vi "Host.vi"() -> ()   [LabVIEW 2018]
uses:
  <vilib>/userdefined/High Color/nirio_resource_hc.ctl
  <instrlib>/niDCPower/nidcpower.llb/niDCPower Measurement Type.ctl
  <vilib>/FPGAPlugInAG/PXI-7953R/niLvFpga_Open_PXI-7953R.vi
  <vilib>/rvi/interface/common/dynamic/niFpgaDynamicAddResources.vi
  <vilib>/FPGAPlugInAG/Dynamic/niLvFpga_Reset_Dynamic.vi
  <vilib>/FPGAPlugInAG/Dynamic/niLvFpga_Run_Dynamic.vi
  <vilib>/Utility/error.llb/Error Cluster From Error Code.vi
  <vilib>/rvi/errors/niLvFpgaAdjustHostInterfaceError.vi
  <vilib>/FPGAPlugInAG/Dynamic/niLvFpga_Abort_Dynamic.vi
  <vilib>/rvi/interface/nirviOpenFPGA/nirviOpenFPGA.xnode
  FPGA Bitfiles/EV76C661_FPGATarget_Target_LxE3WAGXilk.lvbitx
  <vilib>/rvi/interface/nirviMethod/nirviMethod.xnode
  <vilib>/rvi/interface/nirviReadWriteControl/nirviReadWriteControl.xnode
  NiFpgaLv.dll
  <vilib>/rvi/interface/Simulation/niFpgaSimulationCallBeginRW.vi
  <vilib>/FPGAPlugInAG/Dynamic/niLvFpga_ReadFifo_Dynamic.vi
  <vilib>/rvi/errors/niLvFpgaMergeErrorWithErrorCode.vi
panel:
  out "Image":T1(plugin-control)
  in  "Содержание всех регистров":u32[](array[numeric])=[1, 0, 0, 0, 32880, 0, 53338, 2561, 56217, 24976, 512, 260, 0, 0, 512, 0, 0, 0, 6, 1024, 6, 1280, 0, 0, 0, 0, 0, 512, 0, 0, 0, 6, 1024, 6, 1280, 0, 512, 0, 0, 0, 6, 1024, 6, 1280, 0, 512, 0, 0, 0, 6, 1024, 6, 1280, 0, 32896, 32896, 0, 14464, 32960, 0, 0, 0, 0, 0, 0, 0, 0, 0, 8192, 0, 0, 0, 0, 31601, 0, 0, 0, 0, 0, 0, 0, 0, 0, 0, 0, 0, 0, 0, 0, 0, 0, 0, 0, 0, 0, 0, 0, 0, 0, 0, 0, 0, 0, 0, 0, 0, 0, 0, 0, 0, 0, 0, 0, 0, 0, 0, 0, 0, 0, 0, 0, 0, 0, 0, 0, 0, 0, 2048]
  in  "Запись 6 регистров":u32[](array[numeric])=[2561, 56217, 24976, 512, 260, 512]
  in  "SPI_прошить":bool
  out "ST":bool
  in  "RESET":bool
  in  "Автомат":bool
  in  "VDD33_ON":bool
  in  "VDD18_ON":bool
  in  "Светлый (T)\nТемный (F)":bool
  in  "Frames":path=path "C:/LabView_PRJ/EV76C661/FRAMES"
  in  "ПРИМЕЧАНИЕ":string
  in  "SAVE":bool
  in  "Получить кадр":bool
  out "Data":u8[][](array[numeric])
  in  "Непрерывно":bool
  out "Сбои":i32
  out "СБОЙ":string="ОК"
  out "СБОЙ!":bool
  out "ПОСЛЕДНИЙ СБОЙ":string="0"
  out "COUNT":u8
  out "SPI_OUT":bool[](array[boolean])
  in  "МАСКИРУЕМ":i32[](array[numeric])=[0, -1, 2, 3, 4, 5, 6, 7, 8, 9, 10, 11, 12, 13, 14, 15, 16, 17, 18, 19, 20, 21, 22, 23, 24, 25, 26, 27, 28, 29, 30, 31, 32, 33, 34, 35, 36, 37, 38, 39, 40, 41, 42, 43, 44, 45, 46, 47, 48, 49, 50, 51, 52, 53, 54, 55, 56, 57, 58, 59, -1, -1, -1, -1, -1, -1, -1, -1, -1, -1, -1, -1, -1, -1, -1, -1, -1, -1, -1, -1, -1, -1, -1, -1, -1, -1, -1, -1, -1, -1, -1, -1, -1, -1, -1, -1, -1, -1, -1, -1, -1, -1, -1, -1, -1, -1, -1, -1, -1, -1, -1, -1, -1, -1, -1, -1, -1, -1, -1, -1, -1, -1, -1, -1, -1, -1, -1, 127, 0, 0, 0, 0, 0, 0, 0, 0, 0, 0, 0, 0, 0, 0, 0, 0, 0, 0, 0, 0, 0, 0, 0, 0, 0, 0, 0, 0, 0, 0, 0, 0, 0, 0, 0, 0, 0, 0, 0, 0, 0, 0, 0, 0, 0, 0, 0, 0, 0, 0, 0, 0, 0, 0, 0, 0, 0, 0, 0, 0, 0, 0, 0, 0, 0, 0, 0, 0, 0, 0, 0, 0, 0, 0, 0, 0, 0, 0, 0, 0, 0, 0, 0, 0, 0, 0, 0, 0, 0, 0, 0, 0, 0, 0, 0, 0, 0, 0, 0, 0, 0, 0, 0, 0, 0, 0, 0, 0, 0, 0, 0, 0, 0, 0, 0, 0, 0, 0, 0, 0, 0, 0, 0, 0, 0, 0, 0, 0]
  in  "ПРОВЕРКА СБОЕВ?":bool
  out "GC":u8
  out "REG_WR":bool
  in  "SEL_T, мс":u32=100
  in  "SIM_SEL":bool
  out "SEL":bool
  in  "VDD18A_selcur":dbl=0.05 caption="current limit" format="%_6p"
  in  "VDD33A_selcur":dbl=0.05 caption="current limit" format="%_6p"
  in  "VDD18D_selcur":dbl=0.05 caption="current limit" format="%_6p"
  out "VDD18A":i32
  out "VDD18A":bool
  out "VDD33A":i32
  out "VDD33A":bool
  out "VDD18D":i32
  out "VDD18D":bool
  in  "VDD18A, V":dbl=1.8 caption="voltage level" format="%_6p"
  in  "VDD18A_curlim, A":dbl=0.1 caption="current limit" format="%_6p"
  in  "VDD33A_curlim, A":dbl=0.1 caption="current limit" format="%_6p"
  out "VDD18A_cur, A":dbl caption="measurement" format="%_6g"
  out "VDD33A_cur, A":dbl caption="measurement" format="%_6g"
  in  "VDD33A, V":dbl=3.3 caption="voltage level" format="%_6p"
  in  "VDD18D, V":dbl=1.8 caption="voltage level" format="%_6p"
  in  "VDD18D_curlim, A":dbl=0.1 caption="current limit" format="%_6p"
  out "VDD18D_cur, A":dbl caption="measurement" format="%_6g"
  in  "Питание":bool
  out "VDD33A Chart":dbl(graph)=0.0006520018718277456
  out "VDD18D Chart":dbl(graph)=-6.889343232631937
  out "VDD18A Chart":dbl(graph)=0.09491557293549348 caption="Waveform Chart 5"
  in  "Стоп":bool
  in  "VDD18A_33A":refnum<k15>="PXI1Slot2" caption="instrument handle"
  in  "VDD18D":refnum<k15>="PXI1Slot3" caption="instrument handle"
  in  "resource name":T2="PXI1Slot6"
  in  "SEU":path=path "C:/LabView_PRJ/EV76C661/SEU"
  in  "SEL":path=path "C:/LabView_PRJ/EV76C661/SEL"
  out "Номер образца":string="0"
  # "1,6/1,8/2,0"
  # "3,15/3,3/3,45"
  # "h07, h08, h09, h0A, h0B, h0E"
  # "h0E - отвечает за экспозицию\nОт 1 до 65535"
  # "1,6/1,8/2,0"
  # "0"
  # "1"
  # "2"
  # "3"
  # "4"
  # "5"
  # "6"
  # "7"
  # "8"
  # "9"
  # "10"
  # "11"
  # "12"
  # "13"
  # "14"
  # "15"
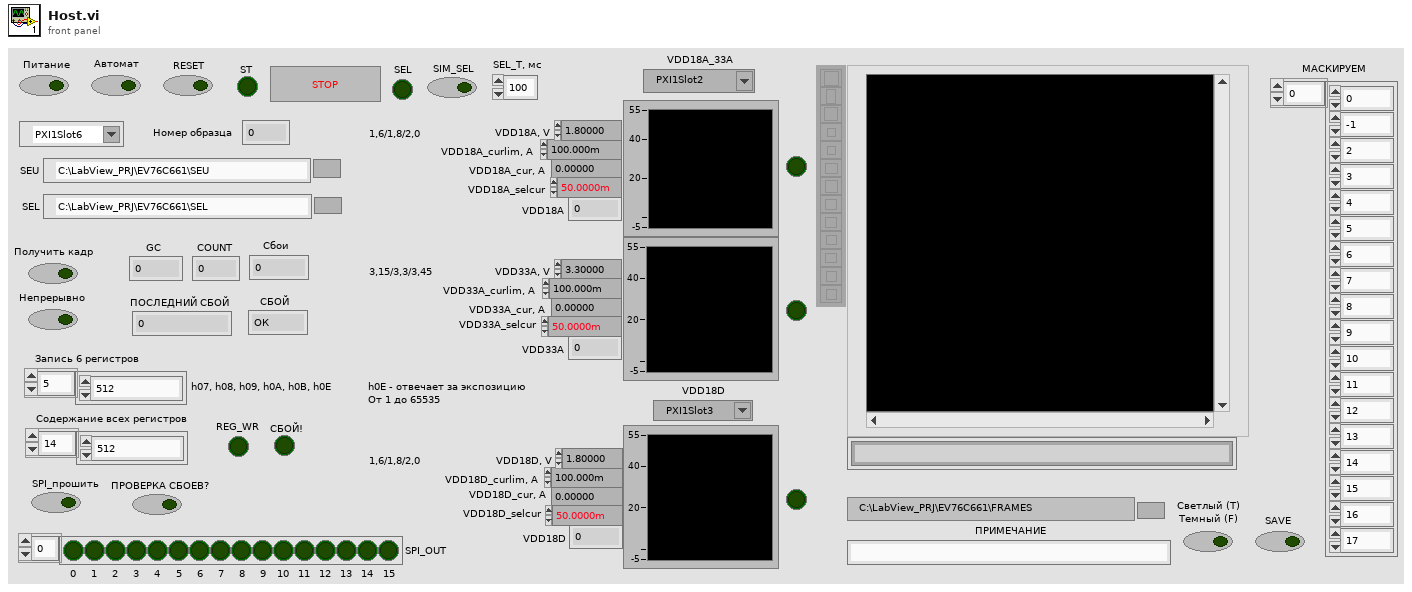
[diagram p1: front panel]
types:
  T1 = typedef "IMAQ Image.ctl" = refnum<image>
  T2 = typedef "nirio_resource_hc.ctl" = tag
  T3 = typedef "Image Type" = u32
  T4 = enum16{"open", "replace", "create", "open or create", "replace or create", "replace or create with confirmation"}
  T5 = typedef "niDCPower Measurement Type.ctl" = i32
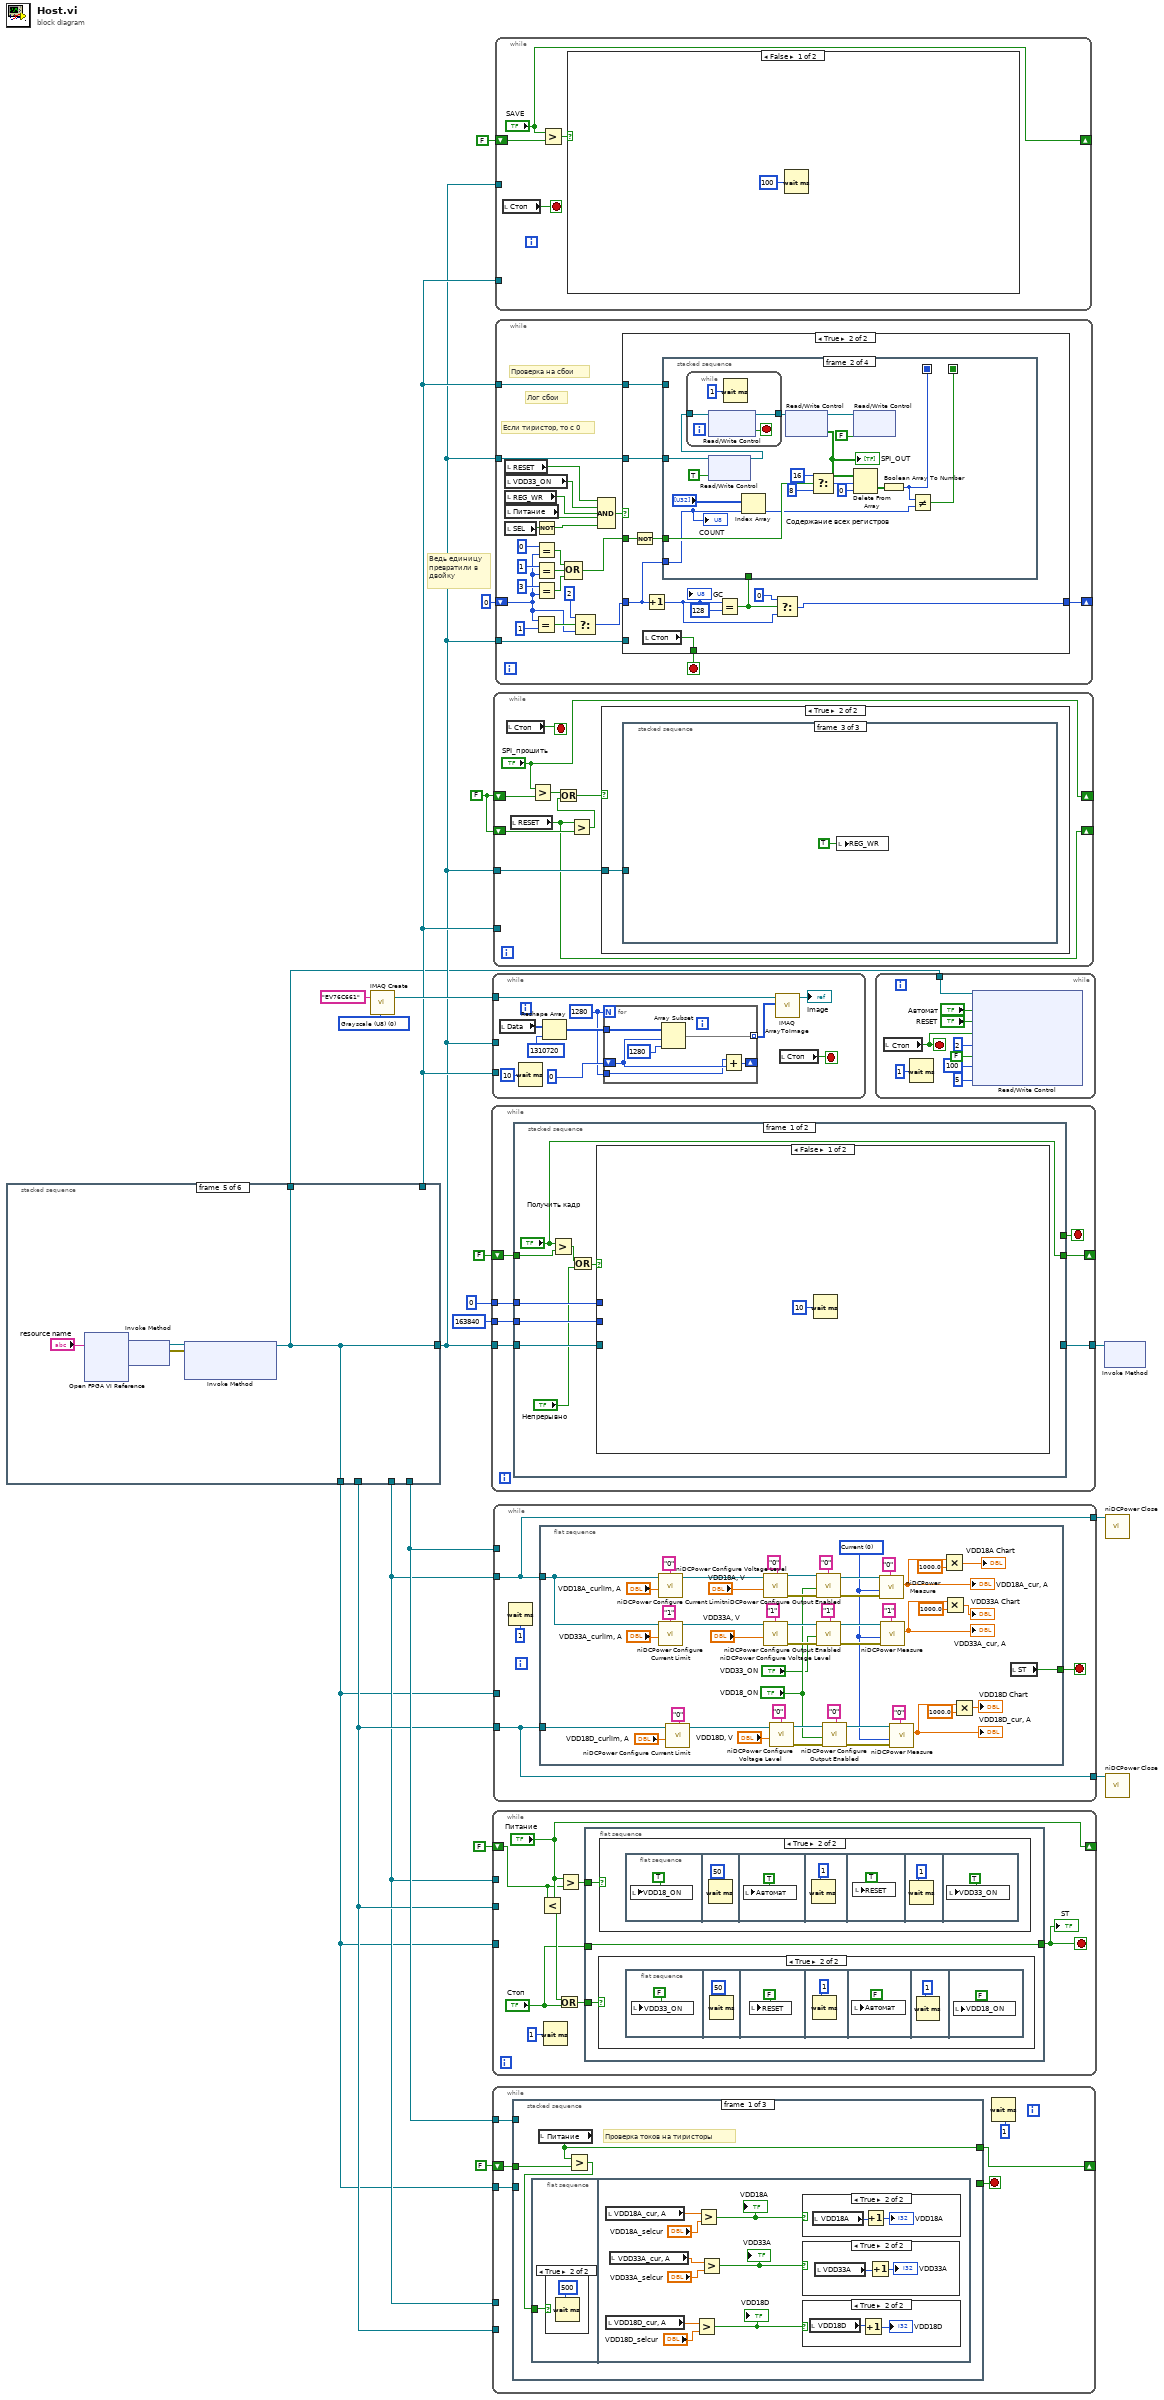
[diagram p0: block diagram]
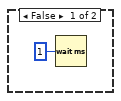
[diagram p2: hidden frame]
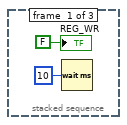
[diagram p3: hidden frame]
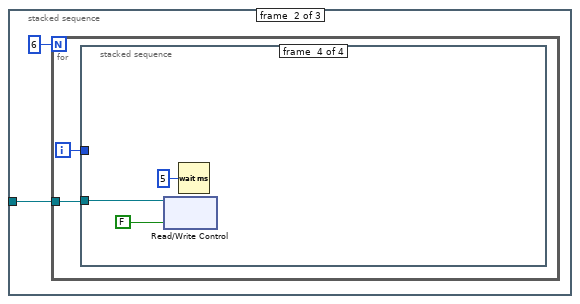
[diagram p4: hidden frame]
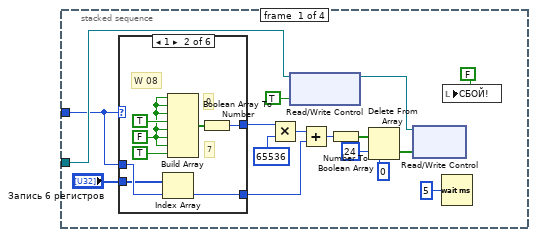
[diagram p5: hidden frame]
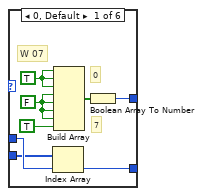
[diagram p6: hidden frame]
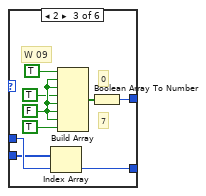
[diagram p7: hidden frame]
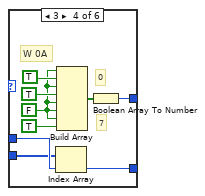
[diagram p8: hidden frame]
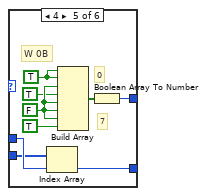
[diagram p9: hidden frame]
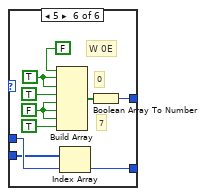
[diagram p10: hidden frame]
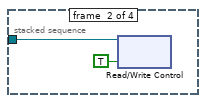
[diagram p11: hidden frame]
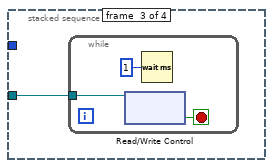
[diagram p12: hidden frame]
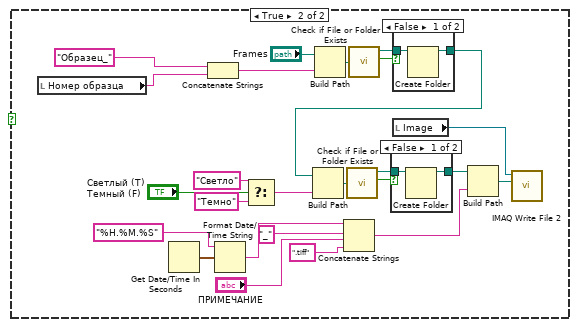
[diagram p15: hidden frame]
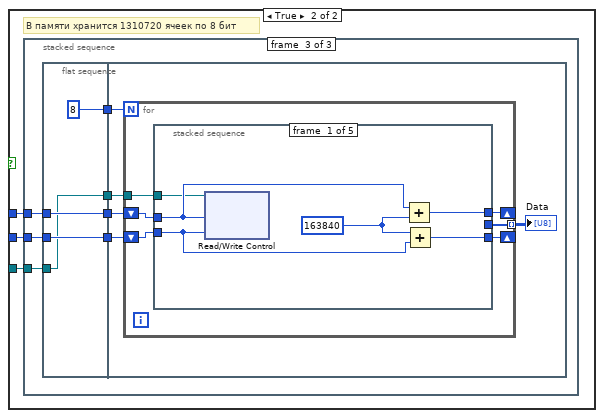
[diagram p18: hidden frame]
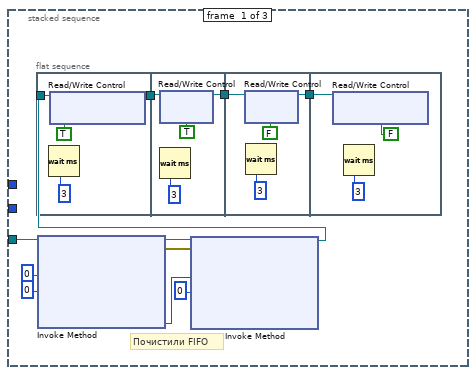
[diagram p19: hidden frame]
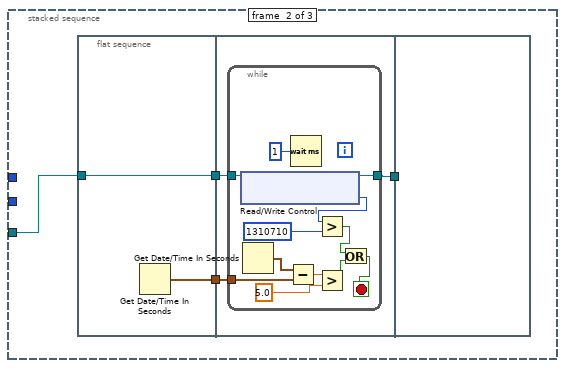
[diagram p20: hidden frame]
diagram:
  w3 = FALSE
  w16 = T3 0 items=["Grayscale (U8)", "Grayscale (I16)", "Grayscale (SGL)", "Complex (CSG)", "RGB (U32)", "HSL (U32)", "RGB (U64)"] ("Image Type")
  # "Ведь единицу \nпревратили в \nдвойку"
  n1 = stacked-sequence {
    tunnel: [_ _ _ _ w92 _] -> w2
    tunnel: [_ _ _ _ _ w99] -> w8
    tunnel: [_ _ _ _ _ w98] -> w7
    tunnel: [_ _ w37 _ _ _] -> w9
    tunnel: [_ _ _ _ w92 _] -> w6
    tunnel: [_ _ _ w63 _ _] -> w5
    tunnel: [_ _ _ _ w92 _] -> w1
    frame #0 {
      n2 = call "Begin.vi"() -> ("Номер образца 2"=→"Номер образца":string)  [unwired: 11 in]
    }
    frame #1 {
      w26 = 0
      w27 = ""
      w23 = FALSE
      n3 = local write "ПОСЛЕДНИЙ СБОЙ"(w27) -> ()
      n4 = local write "СБОЙ"(w27) -> ()
      n5 = local write "Сбои"(w26) -> ()
      n6 = local write "VDD18A"(w26) -> ()
      n7 = local write "VDD33A"(w26) -> ()
      n8 = local write "VDD18D"(w26) -> ()
      n9 = local write "GC"(u8 0 ("GC")) -> ()
      n10 = local write "COUNT"(u16 0 ("COUNT")) -> ()
      n11 = local write "RESET"(w23) -> ()
      n12 = local write "SPI_прошить"(w23) -> ()
      n13 = local write "REG_WR"(w23) -> ()
      n14 = local write "Непрерывно"(w23) -> ()
      n15 = local write "Получить кадр"(w23) -> ()
      n16 = local write "VDD18A"(w23) -> ()
      n17 = local write "VDD33A"(w23) -> ()
      n18 = local write "VDD18D"(w23) -> ()
      n19 = local write "ST"(w23) -> ()
      n20 = local write "SEL"(w23) -> ()
      n21 = local write "Питание"(w23) -> ()
      n22 = local write "Стоп"(w23) -> ()
      n23 = local write "СБОЙ!"(w23) -> ()
      n24 = local write "SAVE"(w23) -> ()
      n25 = local write "ПРОВЕРКА СБОЕВ?"(w23) -> ()
      n26 = local write "Автомат"(w23) -> ()
      n27 = local write "SIM_SEL"(w23) -> ()
      n28 = local write "VDD18_ON"(w23) -> ()
      n29 = local write "VDD33_ON"(w23) -> ()
    }
    frame #2 {
      w38 = "\t"
      # "Инициализаци первой строки лога по токам"
      n30 = local read "Номер образца"() -> (w50:string)
      n31 = Build Path(base path="SEL", name or relative path=w50) -> (appended path=w52:path)
      n32 = Get Date/Time In Seconds() -> (seconds since 1Jan1904=w45:timestamp)
      n33 = call <vilib>:"Check if File or Folder Exists.vi"("path"=w52) -> ("file or folder exists?"=w53:bool, "dup path"=w54:path)  [unwired: 8 in, 1 out]
      n34 = Format Date/Time String(time format string (%c)="%d %H.%M.%S", seconds (now)=w45) -> (date/time string=w42:string)  [unwired: 1 in]
      n35 = case shown="False" w53 {
        tunnel: w54 -> [w60 w61]
        tunnel: [w59 w61] -> w36
        frame False {
          n36 = Create Folder(path (use dialog)=w60) -> (created path=w59:path)  [unwired: 2 in, 2 out]
        }
        frame True {
        }
      }
      n37 = Concatenate Strings(w42, ".xls" ("string")) -> (w40:string)
      n38 = Build Path(base path=w36, name or relative path=w40) -> (appended path=w43:path)
      n39 = Open/Create/Replace File(file path (use dialog)=w43, operation (0:open)=T4."open or create", access (0:read/write)=enum16{"read/write", "read-only", "write-only"}."read/write") -> (refnum out=w46:refnum<file>)  [unwired: 3 in, 2 out]
      n40 = case shown="True" TRUE {
        tunnel: w46 -> [w55 w58]
        tunnel: [w55 w56] -> w39
        frame False {
        }
        frame True {
          n41 = Set File Position(refnum=w58, from (0:start)=enum16{"start", "end", "current"}."end") -> (refnum out=w56:refnum<file>)  [unwired: 2 in, 1 out]
        }
      }
      n42 = Format Into String(initial string=w39, "Time" ("input 1"), w38, "V_18A_cur" ("input 1"), w38, "V_33A_cur" ("input 1"), w38, "V_18D_cur" ("input 1"), w38, "V_18A_sel" ("input 1"), w38, "V_33A_sel" ("input 1"), w38, "V_18D_sel" ("input 1"), "\r\n") -> (resulting string=w37:refnum<file>)  [unwired: 2 in, 1 out]
    }
    frame #3 {
      w72 = "\t"
      n43 = local read "Номер образца"() -> (w80:string)
      n44 = Build Path(base path="SEU", name or relative path=w80) -> (appended path=w82:path)
      n45 = Get Date/Time In Seconds() -> (seconds since 1Jan1904=w78:timestamp)
      n46 = call <vilib>:"Check if File or Folder Exists.vi"("path"=w82) -> ("file or folder exists?"=w83:bool, "dup path"=w84:path)  [unwired: 8 in, 1 out]
      n47 = Format Date/Time String(time format string (%c)="%d %H.%M.%S", seconds (now)=w78) -> (date/time string=w76:string)  [unwired: 1 in]
      n48 = case shown="False" w83 {
        tunnel: w84 -> [w90 w91]
        tunnel: [w89 w91] -> w62
        frame False {
          n49 = Create Folder(path (use dialog)=w90) -> (created path=w89:path)  [unwired: 2 in, 2 out]
        }
        frame True {
        }
      }
      n50 = Concatenate Strings(w76, ".xls" ("string")) -> (w75:string)
      n51 = Build Path(base path=w62, name or relative path=w75) -> (appended path=w77:path)
      n52 = Open/Create/Replace File(file path (use dialog)=w77, operation (0:open)=T4."open or create", access (0:read/write)=enum16{"read/write", "read-only", "write-only"}."read/write") -> (refnum out=w79:refnum<file>)  [unwired: 3 in, 2 out]
      n53 = case shown="True" TRUE {
        tunnel: w79 -> [w85 w88]
        tunnel: [w85 w86] -> w74
        frame False {
        }
        frame True {
          n54 = Set File Position(refnum=w88, from (0:start)=enum16{"start", "end", "current"}."end") -> (refnum out=w86:refnum<file>)  [unwired: 2 in, 1 out]
        }
      }
      n55 = Format Into String(initial string=w74, "Time" ("input 1"), w72, "Count" ("input 3"), w72, "#reg" ("input 5"), "\r\n") -> (resulting string=w63:refnum<file>)  [unwired: 2 in, 1 out]
    }
    frame #4 {
      n56 = xnode "Open FPGA VI Reference"("resource name"="resource name") -> ("FPGA VI Reference Out"=w97:refnum<k20>, "error out"=w95:errorcluster)  [unwired: 1 in]
      n57 = xnode "Invoke Method"("FPGA VI Reference In"=w97, "error in"=w95) -> ("FPGA VI Reference Out"=w94:refnum<k20>, "error out"=w96:errorcluster)
      n58 = xnode "Invoke Method"("FPGA VI Reference In"=w94, "error in"=w96) -> ("FPGA VI Reference Out"=w92:refnum<k20>)  [unwired: 1 in, 1 out]
    }
    frame #5 {
      n59 = call <instrlib>:"niDCPower Initialize.vi"("resource name"="VDD18A_33A") -> ("error out"=w106:errorcluster, "instrument handle out"=w108:refnum<k15>)  [unwired: 3 in, 6 out]
      n60 = call <instrlib>:"niDCPower Initialize.vi"("resource name"="VDD18D") -> ("error out"=w107:errorcluster, "instrument handle out"=w109:refnum<k15>)  [unwired: 3 in, 6 out]
      n61 = call <instrlib>:"niDCPower Configure Voltage Level.vi"("error in (no error)"=w106, "voltage level"=0.0, "channel name"="0,1", "instrument handle"=w108) -> ("instrument handle out"=w98:refnum<k15>)  [unwired: 6 in, 1 out]
      n62 = call <instrlib>:"niDCPower Configure Voltage Level.vi"("error in (no error)"=w107, "voltage level"=0.0, "channel name"="0", "instrument handle"=w109) -> ("instrument handle out"=w99:refnum<k15>)  [unwired: 6 in, 1 out]
    }
  }
  n63 = call "IMAQ Create"("Image Name"="EV76C661", "Image Type"=w16) -> ("New Image"=w15:T1)  [unwired: 3 in, 1 out]
  n64 = while {
    tunnel: w2 -> [w116]
    tunnel: [w115] -> w21
    tunnel: u32 163840 ("163840") -> [w114]
    tunnel: u32 0 -> [w112]
    shift-right: [w110] -> _
    shift-left: FALSE ("Получить кадр") -> [w111]
    stop <- w113 stop-if-true
    n65 = stacked-sequence {
      tunnel: w116 -> [w123 w220]
      tunnel: [_ w220] -> w115
      tunnel: w114 -> [w124 _]
      tunnel: [_ w219] -> w113
      tunnel: w112 -> [w122 _]
      tunnel: w111 -> [w121 _]
      tunnel: ["Получить кадр" _] -> w110
      frame #0 {
        n66 = Greater?(x="Получить кадр", y=w121) -> (0:w120:bool)
        n67 = Or(x=w120, y="Непрерывно") -> (x .or. y?=w118:bool)
        n68 = case shown="False" w118 {
          tunnel: w123 -> [_ w128]
          tunnel: w124 -> [_ w127]
          tunnel: w122 -> [_ w126]
          frame False {
            n69 = Wait (ms)(milliseconds to wait=u32 10) -> ()  [unwired: 1 out]
          }
          frame True {
            # "В памяти хранится 1310720 ячеек по 8 бит"
            n70 = stacked-sequence {
              tunnel: w128 -> [w133 w156 w182]
              tunnel: w127 -> [_ _ w178]
              tunnel: w126 -> [_ _ w180]
              frame #0 {
                # "Почистили FIFO"
                n71 = flat-sequence {
                  tunnel: w131 -> [w143]
                  tunnel: [w140] -> w132
                  tunnel: w132 -> [w145]
                  tunnel: [w144] -> w130
                  tunnel: w130 -> [w151]
                  tunnel: [w150] -> w129
                  tunnel: w129 -> [w154]
                  frame #0 {
                    n72 = Wait (ms)(milliseconds to wait=u32 3) -> ()  [unwired: 1 out]
                    n73 = xnode "Read/Write Control"("FPGA VI Reference In"=w143, "Кадр в память"=TRUE) -> ("FPGA VI Reference Out"=w140:refnum<k20>)  [unwired: 1 in, 1 out]
                  }
                  frame #1 {
                    n74 = xnode "Read/Write Control"("FPGA VI Reference In"=w145, "TRIG"=TRUE ("Кадр в память")) -> ("FPGA VI Reference Out"=w144:refnum<k20>)  [unwired: 1 in, 1 out]
                    n75 = Wait (ms)(milliseconds to wait=u32 3) -> ()  [unwired: 1 out]
                  }
                  frame #2 {
                    n76 = xnode "Read/Write Control"("FPGA VI Reference In"=w151, "TRIG"=FALSE) -> ("FPGA VI Reference Out"=w150:refnum<k20>)  [unwired: 1 in, 1 out]
                    n77 = Wait (ms)(milliseconds to wait=u32 3) -> ()  [unwired: 1 out]
                  }
                  frame #3 {
                    n78 = xnode "Read/Write Control"("FPGA VI Reference In"=w154, "Кадр в память"=FALSE ("Кадр на ПК")) -> ()  [unwired: 1 in, 2 out]
                    n79 = Wait (ms)(milliseconds to wait=u32 3) -> ()  [unwired: 1 out]
                  }
                }
                n80 = xnode "Invoke Method"("FPGA VI Reference In"=w133, "Number of Elements"=u32 0, "Timeout (ms)"=0) -> ("FPGA VI Reference Out"=w139:refnum<k20>, "error out"=w138:errorcluster, "Elements Remaining"=w137:u32)  [unwired: 1 in, 1 out]
                n81 = xnode "Invoke Method"("FPGA VI Reference In"=w139, "error in"=w138, "Number of Elements"=w137, "Timeout (ms)"=0) -> ("FPGA VI Reference Out"=w131:refnum<k20>)  [unwired: 3 out]
              }
              frame #1 {
                n82 = flat-sequence {
                  tunnel: w156 -> [w159]
                  tunnel: [w159] -> w158
                  tunnel: [w160] -> w155
                  tunnel: w158 -> [w163]
                  tunnel: [w162] -> w157
                  tunnel: w155 -> [w161]
                  tunnel: w157 -> [_]
                  frame #0 {
                    n83 = Get Date/Time In Seconds() -> (seconds since 1Jan1904=w160:timestamp)
                  }
                  frame #1 {
                    n84 = while {
                      tunnel: [w174] -> w162
                      tunnel: w163 -> [w173]
                      tunnel: w161 -> [w170]
                      stop <- w165 stop-if-true
                      n85 = xnode "Read/Write Control"("FPGA VI Reference In"=w173) -> ("FPGA VI Reference Out"=w174:refnum<k20>, "Записали адресов"=w164:u32)  [unwired: 1 in, 1 out]
                      n86 = Get Date/Time In Seconds() -> (seconds since 1Jan1904=w171:timestamp)
                      n87 = Subtract(x=w171, y=w170) -> (x-y=w169:dbl)
                      n88 = Wait (ms)(milliseconds to wait=u32 1) -> ()  [unwired: 1 out]
                      n89 = Greater?(x=w164, y=u32 1310710) -> (0:w167:bool)
                      n90 = Greater?(x=w169, y=5.0) -> (0:w166:bool)
                      n91 = Or(x=w167, y=w166) -> (x .or. y?=w165:bool)
                    }
                  }
                  frame #2 {
                  }
                }
              }
              frame #2 {
                n92 = flat-sequence {
                  tunnel: w182 -> [w183]
                  tunnel: [w186] -> w181
                  tunnel: w180 -> [w186]
                  tunnel: [w185] -> w179
                  tunnel: w178 -> [w185]
                  tunnel: [8 ("For FIFO")] -> w177
                  tunnel: [w183] -> w176
                  tunnel: w181 -> [w191]
                  tunnel: w179 -> [w190]
                  tunnel: w177 -> [w189]
                  tunnel: w176 -> [w188]
                  frame #0 {
                  }
                  frame #1 {
                    n93 = for {
                      N: w189 -> [_]
                      shift-right: [w195] -> _
                      shift-left: w191 -> [w197]
                      shift-right: [w194] -> _
                      shift-left: w190 -> [w196]
                      tunnel: w188 -> [w193]
                      tunnel: [w192] -> w187 mode=indexing
                      n94 = stacked-sequence {
                        tunnel: [_ _ _ _ w216] -> w192
                        tunnel: [w203 _ _ _ _] -> w195
                        tunnel: [w202 _ _ _ _] -> w194
                        tunnel: w197 -> [w200 _ _ _ _]
                        tunnel: w196 -> [w201 _ _ _ _]
                        tunnel: w193 -> [w199 w204 w206 w208 w215]
                        frame #0 {
                          w198 = u32 163840 ("163840")
                          n95 = xnode "Read/Write Control"("FPGA VI Reference In"=w199, "Нач_адр"=w200, "Кон_адр"=w201) -> ()  [unwired: 1 in, 2 out]
                          n96 = Add(x=w200, y=w198) -> (x+y=w203:u32)
                          n97 = Add(x=w198, y=w201) -> (x+y=w202:u32)
                        }
                        frame #1 {
                          n98 = xnode "Read/Write Control"("FPGA VI Reference In"=w204, "Кадр на ПК"=TRUE ("HOST")) -> ()  [unwired: 1 in, 2 out]
                        }
                        frame #2 {
                          n99 = xnode "Read/Write Control"("FPGA VI Reference In"=w206, "Кадр на ПК"=FALSE ("HOST")) -> ()  [unwired: 1 in, 2 out]
                        }
                        frame #3 {
                          n100 = while {
                            tunnel: w208 -> [w209]
                            stop <- w211 stop-if-true
                            # "Записан FIFO?"
                            n101 = xnode "Read/Write Control"("FPGA VI Reference In"=w209) -> ("Записали FIFO"=w211:bool)  [unwired: 1 in, 2 out]
                            n102 = Wait (ms)(milliseconds to wait=u32 1) -> ()  [unwired: 1 out]
                          }
                        }
                        frame #4 {
                          n103 = xnode "Invoke Method"("FPGA VI Reference In"=w215, "Number of Elements"=u32 0, "Timeout (ms)"=0) -> ("FPGA VI Reference Out"=w217:refnum<k20>, "Elements Remaining"=w218:u32)  [unwired: 1 in, 2 out]
                          n104 = xnode "Invoke Method"("FPGA VI Reference In"=w217, "Number of Elements"=w218, "Timeout (ms)"=0) -> ("Data"=w216:u8[])  [unwired: 1 in, 3 out]
                        }
                      }
                    }
                    "Data" <- w187
                  }
                }
              }
            }
          }
        }
      }
      frame #1 {
        n105 = local read "Стоп"() -> (w219:bool)
      }
    }
  }
  n106 = while {
    tunnel: w15 -> [w227]
    tunnel: w2 -> [_]
    tunnel: w5 -> [_]
    stop <- w230 stop-if-true
    w221 = 1280 ("length")
    n107 = local read "Data"() -> (w228:u8[][])
    n108 = Wait (ms)(milliseconds to wait=u32 10) -> ()  [unwired: 1 out]
    n109 = Reshape Array(w228, 1310720 ("dimension size")) -> (w225:u8[])
    n110 = for {
      N: w221 -> [_]
      tunnel: w225 -> [w236]
      shift-right: [w235] -> _
      shift-left: 0 ("index") -> [w234]
      tunnel: [w233] -> w223 mode=indexing
      tunnel: w221 -> [w232]
      n111 = Array Subset(array=w236, index=w234, length=1280) -> (w233:u8[])
      n112 = Add(x=w232, y=w234) -> (x+y=w235:i32)
    }
    n113 = call "IMAQ ArrayToImage"("Image Pixels (U8)"=w223, "Image"=w227) -> ("Image Out"=→"Image":T1)  [unwired: 8 in, 1 out]
    n114 = local read "Стоп"() -> (w230:bool)
  }
  n115 = while {
    shift-right: ["Питание"] -> _
    shift-left: FALSE -> [w243]
    tunnel: w6 -> [_]
    tunnel: w8 -> [_]
    tunnel: w7 -> [_]
    stop <- w237 stop-if-true
    n116 = Less?(x="Питание", y=w243) -> (x < y?=w239:bool)
    n117 = Wait (ms)(milliseconds to wait=u32 1) -> ()  [unwired: 1 out]
    n118 = Or(x=w239, y="Стоп") -> (x .or. y?=w240:bool)
    n119 = Greater?(x="Питание", y=w243) -> (0:w242:bool)
    n120 = flat-sequence {
      tunnel: w240 -> [w247]
      tunnel: w242 -> [w246]
      tunnel: [w245] -> w237
      tunnel: "Стоп" -> [w245]
      frame #0 {
        n121 = case shown="True" w247 {
          frame False {
          }
          frame True {
            n122 = flat-sequence {
              frame #0 {
                n123 = local write "VDD33_ON"(FALSE ("VDD18_ON")) -> ()
              }
              frame #1 {
                n124 = Wait (ms)(milliseconds to wait=u32 50) -> ()  [unwired: 1 out]
              }
              frame #2 {
                n125 = local write "RESET"(FALSE ("Автомат")) -> ()
              }
              frame #3 {
                n126 = Wait (ms)(milliseconds to wait=u32 1) -> ()  [unwired: 1 out]
              }
              frame #4 {
                n127 = local write "Автомат"(FALSE ("RESET")) -> ()
              }
              frame #5 {
                n128 = Wait (ms)(milliseconds to wait=u32 1) -> ()  [unwired: 1 out]
              }
              frame #6 {
                n129 = local write "VDD18_ON"(FALSE ("VDD33_ON")) -> ()
              }
            }
          }
        }
        n130 = case shown="True" w246 {
          frame False {
          }
          frame True {
            n131 = flat-sequence {
              frame #0 {
                n132 = local write "VDD18_ON"(TRUE ("VDD18_ON")) -> ()
              }
              frame #1 {
                n133 = Wait (ms)(milliseconds to wait=u32 50) -> ()  [unwired: 1 out]
              }
              frame #2 {
                n134 = local write "Автомат"(TRUE ("Автомат")) -> ()
              }
              frame #3 {
                n135 = Wait (ms)(milliseconds to wait=u32 1) -> ()  [unwired: 1 out]
              }
              frame #4 {
                n136 = local write "RESET"(TRUE ("RESET")) -> ()
              }
              frame #5 {
                n137 = Wait (ms)(milliseconds to wait=u32 1) -> ()  [unwired: 1 out]
              }
              frame #6 {
                n138 = local write "VDD33_ON"(TRUE ("VDD33_ON")) -> ()
              }
            }
          }
        }
      }
    }
    "ST" <- w237
  }
  n139 = while {
    shift-right: [w266] -> _
    shift-left: FALSE -> [w265]
    tunnel: w6 -> [w264]
    tunnel: w9 -> [w263]
    tunnel: w8 -> [_]
    tunnel: w7 -> [_]
    stop <- w262 stop-if-true
    n140 = stacked-sequence {
      tunnel: [w268 _ _] -> w266
      tunnel: w265 -> [w269 _ _]
      tunnel: w264 -> [_ _ _]
      tunnel: w263 -> [_ w300 _]
      tunnel: [_ _ w317] -> w262
      frame #0 {
        # "Проверка токов на тиристоры"
        n141 = flat-sequence {
          tunnel: w270 -> [w271]
          frame #0 {
            n142 = case shown="True" w271 {
              frame False {
              }
              frame True {
                n143 = Wait (ms)(milliseconds to wait=u32 500) -> ()  [unwired: 1 out]
              }
            }
          }
          frame #1 {
            n144 = local read "VDD18A_cur, A"() -> (w275:dbl)
            n145 = local read "VDD18D_cur, A"() -> (w273:dbl)
            n146 = local read "VDD33A_cur, A"() -> (w274:dbl)
            n147 = Greater?(x=w273, y="VDD18D_selcur") -> (0:w276:bool)
            "VDD18D" <- w276
            n148 = Greater?(x=w275, y="VDD18A_selcur") -> (0:w280:bool)
            "VDD18A" <- w280
            n149 = Greater?(x=w274, y="VDD33A_selcur") -> (0:w278:bool)
            "VDD33A" <- w278
            n150 = case shown="True" w280 {
              frame False {
              }
              frame True {
                n151 = local read "VDD18A"() -> (w287:i32)
                n152 = Increment(x=w287) -> (x+1=→"VDD18A":i32)
              }
            }
            n153 = case shown="True" w278 {
              frame False {
              }
              frame True {
                n154 = local read "VDD33A"() -> (w284:i32)
                n155 = Increment(x=w284) -> (x+1=→"VDD33A":i32)
              }
            }
            n156 = case shown="True" w276 {
              frame False {
              }
              frame True {
                n157 = local read "VDD18D"() -> (w283:i32)
                n158 = Increment(x=w283) -> (x+1=→"VDD18D":i32)
              }
            }
          }
        }
        n159 = local read "Питание"() -> (w268:bool)
        n160 = Greater?(x=w268, y=w269) -> (0:w270:bool)
      }
      frame #1 {
        w305 = i16 0 ("width (-)")
        w306 = i16 3 ("width (-)")
        w296 = "\t"
        n161 = local read "VDD18A_cur, A"() -> (w293:dbl)
        n162 = local read "VDD33A_cur, A"() -> (w292:dbl)
        n163 = local read "VDD18D_cur, A"() -> (w291:dbl)
        n164 = local read "VDD18A"() -> (w290:i32)
        n165 = local read "VDD33A"() -> (w289:i32)
        n166 = local read "VDD18D"() -> (w288:i32)
        n167 = Number To Fractional String(number=w293, width (-)=w306, precision (6)=w306) -> (F-format string=w304:string)  [unwired: 1 in]
        n168 = Number To Fractional String(number=w292, width (-)=w306, precision (6)=w306) -> (F-format string=w303:string)  [unwired: 1 in]
        n169 = Number To Fractional String(number=w291, width (-)=w306, precision (6)=w306) -> (F-format string=w302:string)  [unwired: 1 in]
        n170 = Number To Fractional String(number=w290, width (-)=w305, precision (6)=w305) -> (F-format string=w299:string)  [unwired: 1 in]
        n171 = Number To Fractional String(number=w289, width (-)=w305, precision (6)=w305) -> (F-format string=w298:string)  [unwired: 1 in]
        n172 = Number To Fractional String(number=w288, width (-)=w305, precision (6)=w305) -> (F-format string=w297:string)  [unwired: 1 in]
        n173 = Get Date/Time In Seconds() -> (seconds since 1Jan1904=w316:timestamp)
        n174 = Format Date/Time String(time format string (%c)="%d %H:%M:%S:%3u", seconds (now)=w316) -> (date/time string=w307:string)  [unwired: 1 in]
        n175 = local read "VDD33A"() -> (w311:bool)
        n176 = local read "VDD18A"() -> (w310:bool)
        n177 = local read "VDD18D"() -> (w309:bool)
        n178 = local read "SIM_SEL"() -> (w308:bool)
        n179 = Compound Arithmetic op=OR(w311, w310, w309, w308) -> (w301:bool)
        n180 = Select(t="!!!", s=w301, f="") -> (s? t:f=w295:string)
        n181 = Concatenate Strings(w307, w296, w304, w296, w303, w296, w302, w296, w299, w296, w298, w296, w297, w296, w296, w295, "\r\n") -> (w315:string)
        n182 = Format Into String(initial string=w300, w315) -> ()  [unwired: 2 in, 2 out]
      }
      frame #2 {
        n183 = local read "VDD33A"() -> (w322:bool)
        n184 = local read "VDD18A"() -> (w321:bool)
        n185 = local read "VDD18D"() -> (w320:bool)
        n186 = Compound Arithmetic op=OR(w322, w321, w320, "SIM_SEL") -> (w318:bool)
        "SEL" <- w318
        n187 = case shown="True" w318 {
          tunnel: [w323 w324] -> w317
          frame False {
            n188 = local read "Стоп"() -> (w323:bool)
          }
          frame True {
            n189 = flat-sequence {
              tunnel: [w329] -> w324
              frame #0 {
                n190 = local write "Питание"(FALSE ("SYS_RESET")) -> ()
                n191 = local write "REG_WR"(FALSE ("SYS_RESET")) -> ()
              }
              frame #1 {
                n192 = Wait (ms)(milliseconds to wait="SEL_T, мс") -> ()  [unwired: 1 out]
              }
              frame #2 {
                n193 = local write "Питание"(TRUE ("SYS_RESET")) -> ()
              }
              frame #3 {
                n194 = local read "Стоп"() -> (w329:bool)
              }
            }
          }
        }
      }
    }
    n195 = Wait (ms)(milliseconds to wait=u32 1) -> ()  [unwired: 1 out]
  }
  n196 = while {
    tunnel: w8 -> [w330]
    tunnel: w7 -> [w331]
    tunnel: [w331] -> w13
    tunnel: [w330] -> w12
    tunnel: w9 -> [_]
    tunnel: w6 -> [_]
    stop <- w332 stop-if-true
    n197 = Wait (ms)(milliseconds to wait=u32 1) -> ()  [unwired: 1 out]
    n198 = flat-sequence {
      tunnel: w331 -> [w339]
      tunnel: w330 -> [w338]
      tunnel: [w334] -> w332
      frame #0 {
        w349 = T5 0 items=["Current", "Voltage"] ("measurement type")
        n199 = call <instrlib>:"niDCPower Configure Current Limit.vi"("current limit"="VDD18A_curlim, A", "channel name"="0", "instrument handle"=w339) -> ("instrument handle out"=w371:refnum<k15>)  [unwired: 7 in, 1 out]
        n200 = call <instrlib>:"niDCPower Configure Current Limit.vi"("current limit"="VDD33A_curlim, A", "channel name"="1", "instrument handle"=w339) -> ("instrument handle out"=w372:refnum<k15>)  [unwired: 7 in, 1 out]
        n201 = call <instrlib>:"niDCPower Configure Current Limit.vi"("current limit"="VDD18D_curlim, A", "channel name"="0", "instrument handle"=w338) -> ("instrument handle out"=w354:refnum<k15>)  [unwired: 7 in, 1 out]
        n202 = call <instrlib>:"niDCPower Configure Voltage Level.vi"("voltage level"="VDD18A, V", "channel name"="0", "instrument handle"=w371) -> ("error out"=w364:errorcluster, "instrument handle out"=w367:refnum<k15>)  [unwired: 7 in]
        n203 = call <instrlib>:"niDCPower Configure Voltage Level.vi"("voltage level"="VDD33A, V", "channel name"="1", "instrument handle"=w372) -> ("error out"=w365:errorcluster, "instrument handle out"=w366:refnum<k15>)  [unwired: 7 in]
        n204 = call <instrlib>:"niDCPower Configure Voltage Level.vi"("voltage level"="VDD18D, V", "channel name"="0", "instrument handle"=w354) -> ("error out"=w358:errorcluster, "instrument handle out"=w359:refnum<k15>)  [unwired: 7 in]
        n205 = call <instrlib>:"niDCPower Configure Output Enabled.vi"("error in (no error)"=w364, "output enabled"="VDD18_ON", "channel name"="0", "instrument handle"=w367) -> ("error out"=w376:errorcluster, "instrument handle out"=w375:refnum<k15>)  [unwired: 6 in]
        n206 = call <instrlib>:"niDCPower Configure Output Enabled.vi"("error in (no error)"=w365, "output enabled"="VDD33_ON", "channel name"="1", "instrument handle"=w366) -> ("error out"=w377:errorcluster, "instrument handle out"=w378:refnum<k15>)  [unwired: 6 in]
        n207 = call <instrlib>:"niDCPower Configure Output Enabled.vi"("error in (no error)"=w358, "output enabled"="VDD18_ON", "channel name"="0", "instrument handle"=w359) -> ("error out"=w350:errorcluster, "instrument handle out"=w351:refnum<k15>)  [unwired: 6 in]
        n208 = call <instrlib>:"niDCPower Measure.vi"("error in (no error)"=w376, "measurement type"=w349, "channel name"="0", "instrument handle"=w375) -> ("measurement"=w342:dbl)  [unwired: 5 in, 2 out]
        "VDD18A_cur, A" <- w342
        n209 = call <instrlib>:"niDCPower Measure.vi"("error in (no error)"=w377, "measurement type"=w349, "channel name"="1", "instrument handle"=w378) -> ("measurement"=w345:dbl)  [unwired: 5 in, 2 out]
        "VDD33A_cur, A" <- w345
        n210 = call <instrlib>:"niDCPower Measure.vi"("error in (no error)"=w350, "measurement type"=w349, "channel name"="0", "instrument handle"=w351) -> ("measurement"=w343:dbl)  [unwired: 5 in, 2 out]
        "VDD18D_cur, A" <- w343
        n211 = Multiply(x=w342, y=1000.0) -> (x*y=→"VDD18A Chart":dbl)
        n212 = Multiply(x=w345, y=1000.0) -> (x*y=→"VDD33A Chart":dbl)
        n213 = Multiply(x=w343, y=1000.0) -> (x*y=→"VDD18D Chart":dbl)
        n214 = local read "ST"() -> (w334:bool)
      }
    }
  }
  n215 = while {
    tunnel: w2 -> [w389]
    tunnel: w5 -> [_]
    shift-right: ["SPI_прошить"] -> _
    shift-left: w3 -> [w388]
    shift-right: [w382] -> _
    shift-left: w3 -> [w384]
    stop <- w390 stop-if-true
    n216 = local read "Стоп"() -> (w390:bool)
    n217 = local read "RESET"() -> (w382:bool)
    n218 = Greater?(x="SPI_прошить", y=w388) -> (0:w386:bool)
    n219 = Greater?(x=w382, y=w384) -> (0:w383:bool)
    n220 = Or(x=w386, y=w383) -> (x .or. y?=w385:bool)
    n221 = case shown="True" w385 {
      tunnel: w389 -> [_ w392]
      frame False {
        n222 = Wait (ms)(milliseconds to wait=u32 1) -> ()  [unwired: 1 out]
      }
      frame True {
        n223 = stacked-sequence {
          tunnel: w392 -> [_ w395 _]
          frame #0 {
            n224 = Wait (ms)(milliseconds to wait=u32 10) -> ()  [unwired: 1 out]
            "REG_WR" <- FALSE ("Прошили регистры")
          }
          frame #1 {
            n225 = for {
              N: 6 ("Numeric") -> [_]
              tunnel: w395 -> [w397]
              i -> [w398]
              n226 = stacked-sequence {
                tunnel: w397 -> [w401 w468 w470 w474]
                tunnel: w398 -> [w399 _ _ _]
                frame #0 {
                  n227 = case shown="1" w399 {
                    tunnel: [w418 w428 w434 w445 w453 w463] -> w411
                    tunnel: "Запись 6 регистров" -> [w416 w424 w432 w441 w450 w459]
                    tunnel: w399 -> [w417 w425 w433 w442 w451 w460]
                    tunnel: [w415 w423 w431 w440 w449 w458] -> w408
                    frame 0, Default {
                      w420 = FALSE ("element")
                      w419 = TRUE
                      # "W 07"
                      # "0"
                      # "7"
                      n228 = Index Array(array=w416, index=w417) -> (element=w415:u32)
                      n229 = Build Array(w419, w419, w419, w420, w420, w420, w420, TRUE) -> (w422:bool[])
                      n230 = Boolean Array To Number(Boolean array=w422) -> (number=w418:u32)
                    }
                    frame 1 {
                      w426 = FALSE ("element")
                      # "W 08"
                      # "0"
                      # "7"
                      n231 = Index Array(array=w424, index=w425) -> (element=w423:u32)
                      n232 = Build Array(w426, w426, w426, TRUE ("element"), w426, w426, w426, TRUE) -> (w430:bool[])
                      n233 = Boolean Array To Number(Boolean array=w430) -> (number=w428:u32)
                    }
                    frame 2 {
                      w437 = FALSE ("element")
                      # "W 09"
                      # "0"
                      # "7"
                      n234 = Index Array(array=w432, index=w433) -> (element=w431:u32)
                      n235 = Build Array(TRUE, w437, w437, TRUE ("element"), w437, w437, w437, TRUE) -> (w439:bool[])
                      n236 = Boolean Array To Number(Boolean array=w439) -> (number=w434:u32)
                    }
                    frame 3 {
                      w443 = FALSE ("element")
                      # "W 0A"
                      # "0"
                      # "7"
                      n237 = Index Array(array=w441, index=w442) -> (element=w440:u32)
                      n238 = Build Array(w443, TRUE, w443, TRUE ("element"), w443, w443, w443, TRUE) -> (w448:bool[])
                      n239 = Boolean Array To Number(Boolean array=w448) -> (number=w445:u32)
                    }
                    frame 4 {
                      w456 = FALSE ("element")
                      w452 = TRUE
                      # "W 0B"
                      # "0"
                      # "7"
                      n240 = Index Array(array=w450, index=w451) -> (element=w449:u32)
                      n241 = Build Array(w452, w452, w456, TRUE ("element"), w456, w456, w456, TRUE) -> (w457:bool[])
                      n242 = Boolean Array To Number(Boolean array=w457) -> (number=w453:u32)
                    }
                    frame 5 {
                      w466 = FALSE ("element")
                      w461 = TRUE
                      # "W 0E"
                      # "0"
                      # "7"
                      n243 = Build Array(FALSE ("element"), w461, w461, TRUE ("element"), w466, w466, w466, TRUE) -> (w467:bool[])
                      n244 = Index Array(array=w459, index=w460) -> (element=w458:u32)
                      n245 = Boolean Array To Number(Boolean array=w467) -> (number=w463:u32)
                    }
                  }
                  n246 = Multiply(x=w411, y=u32 65536) -> (x*y=w409:u32)
                  n247 = xnode "Read/Write Control"("FPGA VI Reference In"=w401, "8(F)/16(T)"=TRUE) -> ("FPGA VI Reference Out"=w400:refnum<k20>)  [unwired: 1 in, 1 out]
                  n248 = Add(x=w409, y=w408) -> (x+y=w407:u32)
                  n249 = Number To Boolean Array(number=w407) -> (Boolean array=w406:bool[])
                  n250 = Delete From Array(array=w406, length=24, index=0) -> (deleted portion=w403:bool[])  [unwired: 1 out]
                  n251 = xnode "Read/Write Control"("FPGA VI Reference In"=w400, "MOSI"=w403) -> ()  [unwired: 1 in, 2 out]
                  n252 = Wait (ms)(milliseconds to wait=u32 5) -> ()  [unwired: 1 out]
                  n253 = local write "СБОЙ!"(FALSE ("СБОЙ!")) -> ()
                }
                frame #1 {
                  n254 = xnode "Read/Write Control"("FPGA VI Reference In"=w468, "SPI"=TRUE) -> ()  [unwired: 1 in, 2 out]
                }
                frame #2 {
                  n255 = while {
                    tunnel: w470 -> [w473]
                    stop <- w472 stop-if-true
                    n256 = xnode "Read/Write Control"("FPGA VI Reference In"=w473) -> ("SPI_OFF"=w472:bool)  [unwired: 1 in, 2 out]
                    n257 = Wait (ms)(milliseconds to wait=u32 1) -> ()  [unwired: 1 out]
                  }
                }
                frame #3 {
                  n258 = xnode "Read/Write Control"("FPGA VI Reference In"=w474, "SPI"=FALSE) -> ()  [unwired: 1 in, 2 out]
                  n259 = Wait (ms)(milliseconds to wait=u32 5) -> ()  [unwired: 1 out]
                }
              }
            }
          }
          frame #2 {
            n260 = local write "REG_WR"(TRUE ("REG_WR")) -> ()
          }
        }
      }
    }
  }
  n261 = while {
    shift-right: ["SAVE"] -> _
    shift-left: FALSE ("SAVE") -> [w480]
    tunnel: w5 -> [_]
    tunnel: w2 -> [_]
    stop <- w481 stop-if-true
    n262 = local read "Стоп"() -> (w481:bool)
    n263 = Greater?(x="SAVE", y=w480) -> (0:w479:bool)
    n264 = case shown="False" w479 {
      frame False {
        n265 = Wait (ms)(milliseconds to wait=u32 100) -> ()  [unwired: 1 out]
      }
      frame True {
        n266 = local read "Номер образца"() -> (w487:string)
        n267 = Get Date/Time In Seconds() -> (seconds since 1Jan1904=w502:timestamp)
        n268 = Concatenate Strings("Образец_" ("string"), w487) -> (w485:string)
        n269 = Format Date/Time String(time format string (%c)="%H.%M.%S", seconds (now)=w502) -> (date/time string=w506:string)  [unwired: 1 in]
        n270 = Select(t="Светло", s="Светлый (T)\nТемный (F)", f="Темно") -> (s? t:f=w503:string)
        n271 = Build Path(base path="Frames", name or relative path=w485) -> (appended path=w497:path)
        n272 = Concatenate Strings(w506, "_", "ПРИМЕЧАНИЕ", ".tiff" ("element")) -> (w505:string)
        n273 = call <vilib>:"Check if File or Folder Exists.vi"("path"=w497) -> ("file or folder exists?"=w496:bool, "dup path"=w495:path)  [unwired: 8 in, 1 out]
        n274 = case shown="False" w496 {
          tunnel: w495 -> [w512 w513]
          tunnel: [w511 w513] -> w484
          frame False {
            n275 = Create Folder(path (use dialog)=w512) -> (created path=w511:path)  [unwired: 2 in, 2 out]
          }
          frame True {
          }
        }
        n276 = Build Path(base path=w484, name or relative path=w503) -> (appended path=w498:path)
        n277 = call <vilib>:"Check if File or Folder Exists.vi"("path"=w498) -> ("file or folder exists?"=w499:bool, "dup path"=w500:path)  [unwired: 8 in, 1 out]
        n278 = case shown="False" w499 {
          tunnel: w500 -> [w509 w510]
          tunnel: [w508 w510] -> w504
          frame False {
            n279 = Create Folder(path (use dialog)=w509) -> (created path=w508:path)  [unwired: 2 in, 2 out]
          }
          frame True {
          }
        }
        n280 = local read "Image"() -> (w489:T1)
        n281 = Build Path(base path=w504, name or relative path=w505) -> (appended path=w501:path)
        n282 = call-poly "IMAQ Write File 2"("File Path"=w501, "Image"=w489) -> ()  [unwired: 8 in, 2 out]
      }
    }
  }
  n283 = while {
    tunnel: w2 -> [w534]
    tunnel: w5 -> [w536]
    shift-right: [w537] -> _
    shift-left: u8 0 -> [w516]
    tunnel: w2 -> [w533]
    stop <- w535 stop-if-true
    # "Лог сбои"
    # "Проверка на сбои"
    # "Если тиристор, то с 0"
    n284 = local read "RESET"() -> (w514:bool)
    n285 = local read "VDD33_ON"() -> (w515:bool)
    n286 = local read "REG_WR"() -> (w529:bool)
    n287 = local read "Питание"() -> (w528:bool)
    n288 = local read "SEL"() -> (w527:bool)
    n289 = Equal?(x=w516, y=u8 1 ("x")) -> (x = y?=w519:bool)
    n290 = Not(x=w527) -> (.not. x?=w526:bool)
    n291 = Equal?(x=u8 0, y=w516) -> (x = y?=w532:bool)
    n292 = Equal?(x=u8 1, y=w516) -> (x = y?=w531:bool)
    n293 = Equal?(x=u8 3, y=w516) -> (x = y?=w530:bool)
    n294 = Compound Arithmetic op=OR(w532, w531, w530) -> (w522:bool)
    n295 = Select(t=u8 2, s=w519, f=w516) -> (s? t:f=w518:u8)
    n296 = Compound Arithmetic op=AND(w514, w515, w529, w528, w526) -> (w521:bool)
    n297 = case shown="True" w521 {
      tunnel: w518 -> [_ w541]
      tunnel: [u8 0 w550] -> w537
      tunnel: w534 -> [_ w545]
      tunnel: w536 -> [_ w546]
      tunnel: [w539 w548] -> w535
      tunnel: w533 -> [_ _]
      tunnel: w522 -> [_ w542]
      frame False {
        n298 = local read "Стоп"() -> (w539:bool)
        n299 = Wait (ms)(milliseconds to wait=u32 1) -> ()  [unwired: 1 out]
      }
      frame True {
        n300 = Not(x=w542) -> (.not. x?=w543:bool)
        n301 = local read "Стоп"() -> (w548:bool)
        n302 = Increment(x=w541) -> (x+1=w549:u8)
        "GC" <- w549
        n303 = Equal?(x=w549, y=u8 128) -> (x = y?=w544:bool)
        n304 = stacked-sequence {
          seq-local: [_ w569 _ _] -> [_ _ w592 _]
          seq-local: [_ w568 _ _] -> [_ _ w587 _]
          tunnel: w543 -> [w554 w575 _ _]
          tunnel: w546 -> [_ _ _ w614]
          tunnel: w545 -> [w556 w566 _ _]
          tunnel: w544 -> [_ _ _ w613]
          tunnel: w541 -> [w552 w564 w586 _]
          frame #0 {
            n305 = Select(t=u32 65536 ("y"), s=w554, f=u32 256 ("y")) -> (s? t:f=w562:u32)
            n306 = Multiply(x=w552, y=w562) -> (x*y=w563:u32)
            n307 = Number To Boolean Array(number=w563) -> (Boolean array=w561:bool[])
            n308 = xnode "Read/Write Control"("FPGA VI Reference In"=w556, "8(F)/16(T)"=w554) -> ("FPGA VI Reference Out"=w555:refnum<k20>)  [unwired: 1 in, 1 out]
            n309 = xnode "Read/Write Control"("FPGA VI Reference In"=w555, "MOSI"=w561) -> ("FPGA VI Reference Out"=w553:refnum<k20>)  [unwired: 1 in, 1 out]
            n310 = Wait (ms)(milliseconds to wait=u32 1) -> ()  [unwired: 1 out]
            n311 = xnode "Read/Write Control"("FPGA VI Reference In"=w553, "SPI"=TRUE) -> ()  [unwired: 1 in, 2 out]
          }
          frame #1 {
            n312 = xnode "Read/Write Control"("FPGA VI Reference In"=w566, "SPI"=TRUE) -> ("FPGA VI Reference Out"=w565:refnum<k20>)  [unwired: 1 in, 1 out]
            n313 = while {
              tunnel: w565 -> [w585]
              tunnel: [w583] -> w579
              stop <- w584 stop-if-true
              n314 = xnode "Read/Write Control"("FPGA VI Reference In"=w585) -> ("FPGA VI Reference Out"=w583:refnum<k20>, "SPI_OFF"=w584:bool)  [unwired: 1 in, 1 out]
              n315 = Wait (ms)(milliseconds to wait=u32 1) -> ()  [unwired: 1 out]
            }
            n316 = Index Array(array="Содержание всех регистров", index=w564) -> (element=w570:u32)
            n317 = xnode "Read/Write Control"("FPGA VI Reference In"=w579) -> ("FPGA VI Reference Out"=w581:refnum<k20>, "MISO"=w577:bool[])  [unwired: 1 in, 1 out]
            "SPI_OUT" <- w577
            n318 = Select(t=16, s=w575, f=8) -> (s? t:f=w572:i32)
            n319 = xnode "Read/Write Control"("FPGA VI Reference In"=w581, "SPI"=FALSE) -> ()  [unwired: 1 in, 2 out]
            n320 = Delete From Array(array=w577, length=w572, index=0) -> (deleted portion=w571:bool[])  [unwired: 1 out]
            n321 = Boolean Array To Number(Boolean array=w571) -> (number=w568:u16)
            n322 = Not Equal?(x=w568, y=w570) -> (x != y?=w569:bool)
            "COUNT" <- w564
          }
          frame #2 {
            n323 = Search 1D Array(1D array="МАСКИРУЕМ", element=w586, start index (0)=0) -> (index of element=w596:i32)
            n324 = local read "SEL"() -> (w597:bool)
            n325 = Greater?(x=w596, y=-1) -> (0:w589:bool)
            n326 = Not(x=w597) -> (.not. x?=w590:bool)
            n327 = Compound Arithmetic op=AND(w592, "ПРОВЕРКА СБОЕВ?", w590, w589) -> (w588:bool)
            n328 = case shown="True" w588 {
              tunnel: w586 -> [_ w603]
              tunnel: w587 -> [_ w602]
              frame False {
                n329 = local write "СБОЙ"("ОК" ("Где сбой")) -> ()
              }
              frame True {
                w599 = " " ("string")
                w608 = i16 0 ("width (-)")
                w609 = i16 0 ("width (-)")
                n330 = local read "Сбои"() -> (w611:i32)
                n331 = Number To Fractional String(number=w603, width (-)=w609, precision (6)=w609) -> (F-format string=w606:string)  [unwired: 1 in]
                n332 = Number To Fractional String(number=w602, width (-)=w608, precision (6)=w608) -> (F-format string=w600:string)  [unwired: 1 in]
                n333 = Increment(x=w611) -> (x+1=→"Сбои":i32)
                n334 = Concatenate Strings("#" ("string"), w606, w599, "=" ("string"), w599, w600) -> (→"СБОЙ" →"ПОСЛЕДНИЙ СБОЙ":string)
                "СБОЙ!" <- TRUE ("СБОЙ!")
              }
            }
          }
          frame #3 {
            w619 = i16 0 ("width (-)")
            w618 = "\t"
            # "Пишет, в каком регистре произошел сбой"
            n335 = local read "СБОЙ!"() -> (w612:bool)
            n336 = local read "Сбои"() -> (w622:i32)
            n337 = And(x=w612, y=w613) -> (x .and. y?=w615:bool)
            n338 = case shown="True" w615 {
              frame False {
              }
              frame True {
                n339 = flat-sequence {
                  frame #0 {
                    n340 = local write "RESET"(FALSE ("RESET")) -> ()
                  }
                  frame #1 {
                    n341 = Wait (ms)(milliseconds to wait=u32 2) -> ()  [unwired: 1 out]
                  }
                  frame #2 {
                    n342 = local write "RESET"(TRUE ("RESET")) -> ()
                    n343 = Wait (ms)(milliseconds to wait=u32 5) -> ()  [unwired: 1 out]
                  }
                }
              }
            }
            n344 = Number To Fractional String(number=w622, width (-)=w619, precision (6)=w619) -> (F-format string=w621:string)  [unwired: 1 in]
            n345 = Get Date/Time In Seconds() -> (seconds since 1Jan1904=w625:timestamp)
            n346 = local read "СБОЙ"() -> (w620:string)
            n347 = Format Date/Time String(time format string (%c)="%d %H:%M:%S:%3u", seconds (now)=w625) -> (date/time string=w624:string)  [unwired: 1 in]
            n348 = Concatenate Strings(w624, w618, w621, w618, w620, "\r\n") -> (w623:string)
            n349 = Format Into String(initial string=w614, w623) -> ()  [unwired: 2 in, 2 out]
          }
        }
        n350 = Select(t=u8 0, s=w544, f=w549) -> (s? t:f=w550:u8)
      }
    }
  }
  n351 = while {
    tunnel: w1 -> [w637]
    stop <- w633 stop-if-true
    n352 = local read "Стоп"() -> (w633:bool)
    n353 = Wait (ms)(milliseconds to wait=u32 1) -> ()  [unwired: 1 out]
    n354 = xnode "Read/Write Control"("FPGA VI Reference In"=w637, "Автомат"="Автомат", "RESET"="RESET", "Стоп"=w633, "Делитель (24/? = F, Гц)"=u8 2, "Направление бит"=FALSE, "TRIG_2"=u8 100, "TRIG_1"=u8 5) -> ()  [unwired: 1 in, 2 out]
  }
  n355 = xnode "Invoke Method"("FPGA VI Reference In"=w21) -> ()  [unwired: 1 in, 2 out]
  n356 = call <instrlib>:"niDCPower Close.vi"("instrument handle"=w13) -> ()  [unwired: 10 in, 1 out]
  n357 = call <instrlib>:"niDCPower Close.vi"("instrument handle"=w12) -> ()  [unwired: 10 in, 1 out]
